vi "DBTester4.vi"() -> ()   [LabVIEW 2015]
uses:
  BERTTA.dll
panel:
  in  "col":i32
  out "values":dbl[](array[numeric])
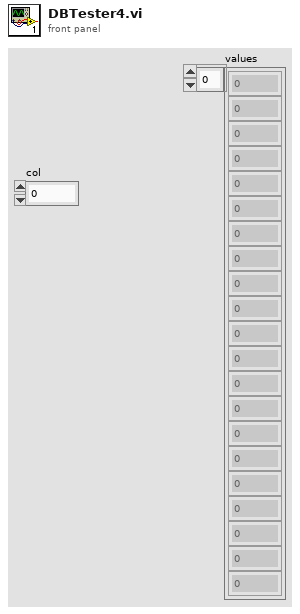
[diagram p1: front panel]
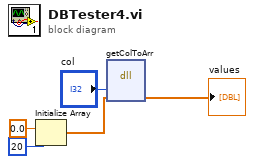
[diagram p0: block diagram]
diagram:
  n1 = Initialize Array(0.0 ("element"), 20 ("dimension size")) -> (w5:dbl[])
  n2 = dll-call lib="C:/Users/xlaraser/Documents/Visual Studio 2017/Projects/Bertta/BERTTA/Debug/BERTTA.dll" fn="getColToArr"("col"="col", "values"=w5) -> ("values"=→"values":dbl[])  [unwired: 5 in, 2 out]
